vi "Close Configuration Reference.vi"(8 "error in (no error)":errorcluster, 11 "Configuration Reference":refnum<data-value>) -> (0 "error out":errorcluster)   [LabVIEW 2020, in "Configuration.lvlib" / "ConfigurationReference.lvclass"]
uses:
  <vilib>/gpm_packages/@cs/Configuration/Source/ConfigurationReference/ConfigurationReference.lvclass
  <vilib>/gpm_packages/@cs/Configuration/Source/ConfigurationReference/ConfigurationReference.lvclass/ConfigurationReference.ctl
  <vilib>/gpm_packages/@cs/Configuration/Source/IConfiguration/IConfiguration.lvclass
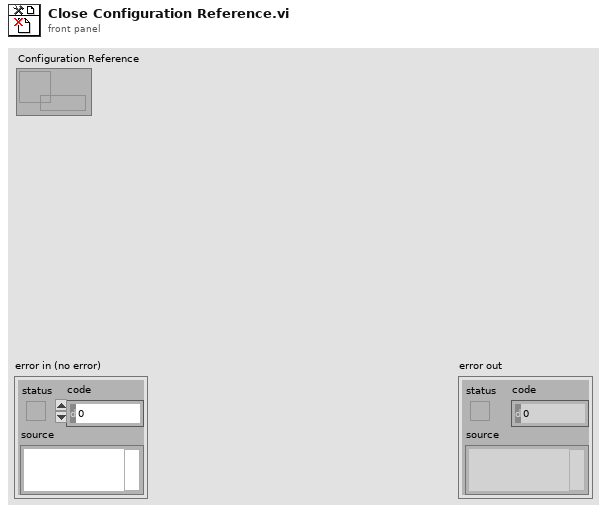
[diagram p1: front panel]
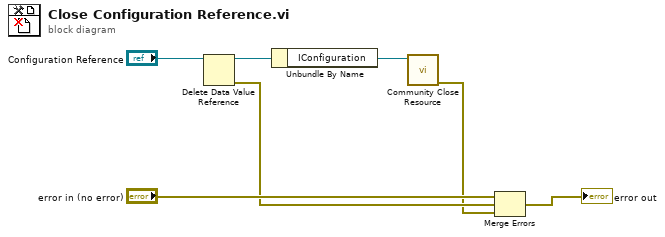
[diagram p0: block diagram]
diagram:
  n1 = Delete Data Value Reference(data value reference="Configuration Reference") -> (data value=w5:refnum<class "ConfigurationReference.lvclass">, error out=w2:errorcluster)  [unwired: 1 in]
  n2 = Unbundle By Name(w5) -> ("IConfiguration"=w4:refnum<class "IConfiguration.lvclass">)
  n3 = call <vilib>:"Community Close Resource.vi"("IConfiguration in"=w4) -> ("error out"=w1:errorcluster)  [unwired: 9 in, 1 out]
  n4 = Merge Errors("error in (no error)", w2, w1) -> (→"error out":errorcluster)
